vi "zmq_check_term.vi"(2 "drop term? (T)":bool=TRUE, 3 "error in":errorcluster) -> (0 "term?":bool, 1 "error out":errorcluster)   [LabVIEW 2020, in "zeromq.lvlib"]
doc: "Checks the input error cluster to see whether the error was ETERM, and optionally removes it. If ETERM is raised, then the socket should be closed immediately.\n\nDetailed API documentation: http://api.zeromq.org/3-2:zmq-ctx-destroy"
uses:
  zeromq.lvlib
panel:
  # "ØMQ"
  # "labview"
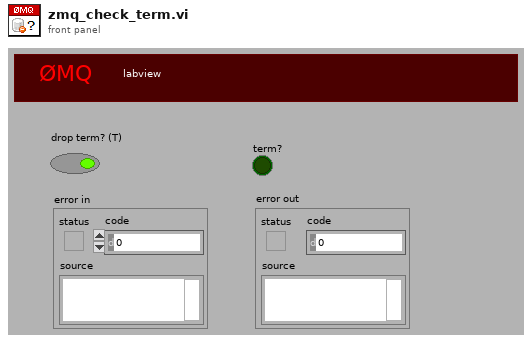
[diagram p1: front panel]
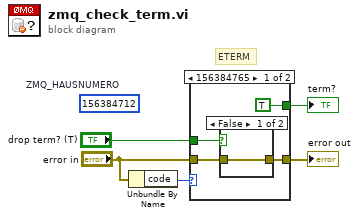
[diagram p0: block diagram]
diagram:
  (unwired) 156384712  # ZMQ_HAUSNUMERO
  # "ETERM"
  n1 = Unbundle By Name("error in") -> ("code"=w2:i32)
  n2 = case shown="156384765" w2 {
    tunnel: [w6 w11] -> w5
    tunnel: "error in" -> [w7 w11]
    tunnel: [TRUE _] -> w4
    tunnel: "drop term? (T)" -> [w8 _]
    frame 156384765 {
      n3 = case shown="False" w8 {
        tunnel: w7 -> [w10 _]
        tunnel: [w10 _] -> w6
        frame False {
        }
        frame True {
        }
      }
    }
    frame Default {
    }
  }
  "error out" <- w5
  "term?" <- w4
